vi "Write Frame.vi"(8 "error in (no error)":errorcluster, 9 "Frame Number":u32, 10 "Frame":u16[][](array[numeric]), 11 "TIFF in":refnum<class "TIFF.lvclass">) -> (0 "error out":errorcluster, 3 "TIFF out":refnum<class "TIFF.lvclass">)   [LabVIEW 2018]
uses:
  TIFF.lvclass
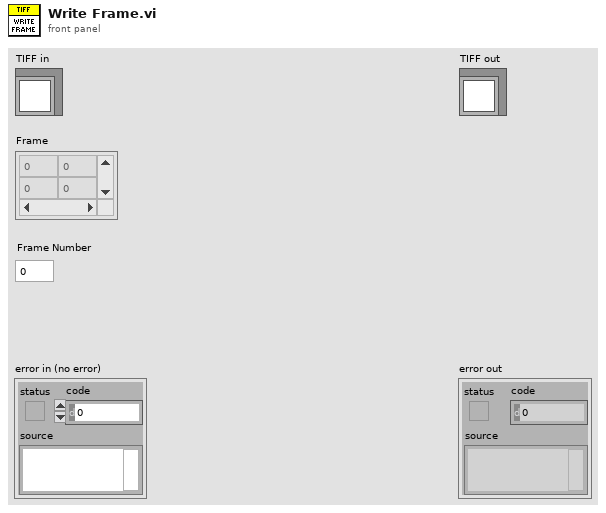
[diagram p1: front panel]
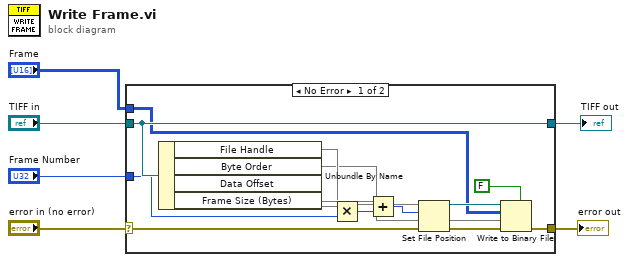
[diagram p0: block diagram]
diagram:
  n1 = case shown="No Error" "error in (no error)" {
    selector: "error in (no error)" -> [w14 w22]
    tunnel: [w12 w22] -> w5
    tunnel: [w20 w21] -> w3
    tunnel: "TIFF in" -> [w20 w21]
    tunnel: "Frame" -> [w8 _]
    tunnel: "Frame Number" -> [w16 _]
    frame No Error {
      n2 = Unbundle By Name(w20) -> ("File Handle"=w10, "Byte Order"=w9, "Data Offset"=w19, "Frame Size (Bytes)"=w17)
      n3 = Multiply(x=w17, y=w16) -> (x*y=w18:u32)
      n4 = Add(x=w19, y=w18) -> (x+y=w15:u32)
      n5 = Set File Position(offset (in bytes) (0)=w15, refnum=w10, error in=w14) -> (refnum out=w11:refnum<file>, error out=w13:errorcluster)  [unwired: 1 in]
      n6 = Write to Binary File(file (use dialog)=w11, data=w8, error in=w13, 5:FALSE ("prepend array or string size? (T)"), 9:w9) -> (error out=w12:errorcluster)  [unwired: 1 in, 2 out]
    }
    frame Error {
    }
  }
  "error out" <- w5
  "TIFF out" <- w3
